vi "GM Count.vi"(0 "QUIT":refnum<vi>, 1 "Scan in Progress":refnum<vi>, 2 "GM1 Measure":refnum<vi>, 3 "Error":refnum<vi>, 4 "Measure GM2":refnum<vi>, 5 "VA Volts":refnum<vi>, 6 "VB Volts":refnum<vi>, 7 "Set Voltage A":refnum<vi>, 8 "GM1 Dwell":refnum<vi>, 9 "Set Voltage B":refnum<vi>, 10 "GM1 LLD":refnum<vi>, 12 "GM1 ULD":refnum<vi>, 14 "GM1 Counts":refnum<vi>, 16 "Emergency":refnum<vi>, 18 "GM2 Dwell":refnum<vi>, 20 "GM2 Counts":refnum<vi>) -> ()   [LabVIEW 2018]
uses:
  <vilib>/Utility/error.llb/DialogType.ctl
  <vilib>/Analysis/baseanly.llb/Mean (DBL).vi
  <vilib>/Analysis/NI_AALBase.lvlib
panel:
  out "Data":u32[](graph)
  out "GM2 Storage":dbl[](array[numeric])
  out "GM1 Storage":dbl[](array[numeric])
  in  "GM Count":T1(tab)
  out "Status B LED":bool
  out "Status A LED":bool
  in  "VB Local":dbl
  out "VB Feedback":dbl caption="(V)"
  out "VA Feedback":dbl caption="(V)"
  in  "VA Local":dbl caption="(V)"
  in  "GM2 Dwell Local":dbl=1.0 caption="Dwell" min=0.1
  in  "GM1 ULD":dbl caption="Upper Limit" max=12.0
  in  "GM1 Dwell Local":dbl=1.0 caption="Dwell" min=0.1
  in  "LLD Right":dbl caption="Lower Limit" max=12.0
  in  "GM2 Threshold":dbl caption="Threshold" min=0.0 max=10000.0 step=10.0
  in  "GM1 Threshold":dbl caption="Threshold" min=0.0 max=10000.0 step=10.0
  out "GM2 Counts Local":i32 caption="Total Counts"
  out "GM2 Rate":dbl caption="Count Rate"
  out "GM2 Average":dbl caption="Average Rate"
  out "Status A":string caption="Device Status Response"
  out "Status B":string caption="Device Status Response"
  out "GM1 Counts Local":i32 caption="Total Counts"
  out "GM1 Rate":dbl caption="Count Rate"
  out "GM1 Average":dbl caption="Average Rate"
  in  "Voltage Error Tolerance":dbl=2.0 caption="V"
  in  "Wait Time":dbl=10.0 caption="s"
  in  "VA Ramp":dbl=30.0 caption="A" min=2.0 step=1.0
  in  "Number of Rates\nto Average":u32=20 min=1 max=1024
  in  "GM1 Spectrum":i32=2 caption="Detector 1"
  in  "GM2 Spectrum":i32=3 caption="Detector 2"
  in  "NHQ 203M Voltage Supply":refnum<visa-resource-name>="COM8"
  out "VA Ramp Feedback":dbl=2.0 caption="V/s" format="%.2f"
  out "Voltage Change Response A":string caption="Voltage Change Response"
  out "Voltage Change Response B":string
  out "VB Ramp Feedback":dbl=2.0 caption="V/s" format="%.2f"
  in  "VB Ramp":sgl=30.0 caption="B" min=2 max=255 step=1
  in  "Feedback Delay":u32=50
  # "Note that the Average Rate is found by simply averaging the last 'n' acquired count rates.  Therefore,\nit may not be an accurate measure of the real count rate in Hz if Dwell has recently been changed."
  # "Detector 1"
  # "Detector 2"
  # "s"
  # "s"
  # "Hz"
  # "Hz"
  # "V"
  # "Hz"
  # "V"
  # "Hz"
  # "mV"
  # "mV"
  # "Voltage Supply B"
  # "Voltage Supply A"
  # "A"
  # "B"
  # "MCA 4 Spectrum #"
  # "NHQ 203 M Ramp Speed"
  # "Sometimes the power supply has trouble getting the actual voltage to the setpoint, especially for low voltages.  This can risk hanging up a scan, which waits for the voltage to reach the setpoint before allowing the next step to occur.  To avoid this problem, the VI will progress the scan if the difference between the actual voltage and the setpoint is less than <Voltage Error Tolerance> AND <Wait Time> has elapsed."
  # "The VI waits for <Feedback Delay> ms between submitting the change voltage command and then checking the state of the power supply."
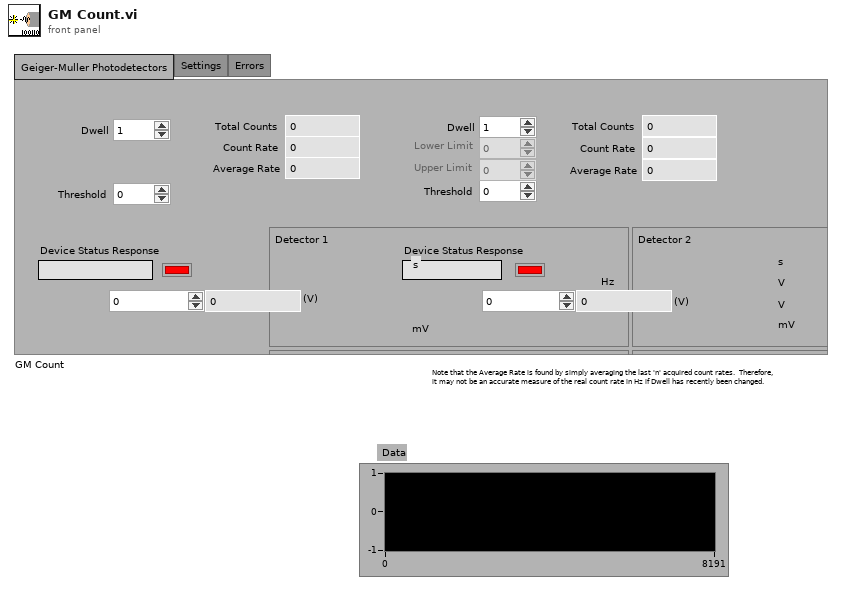
[diagram p1: front panel]
types:
  T1 = enum32{"Geiger-Muller Photodetectors", "Settings", "Errors"}
  T2 = typedef "DialogType.ctl" = u16
  T3 = typedef "iseg NHQ VISA Control.ctl" = cluster{"VISA Resource Name":refnum<visa-resource-name>, "FP Notation":bool, "Maximum Voltage":u32, "Maximum Current":u32}
  T4 = cluster{"Started":u32, "Maxval":u32, "Livetime":dbl, "Deadtime (%)":dbl, "Totalsum":dbl, "ROIsum":dbl, "ROIrate":dbl, "Realtime":dbl, "Netsum":dbl, "Counts":dbl}
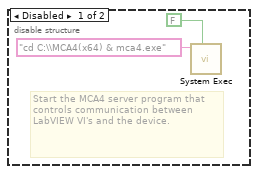
[diagram p2: hidden frame]
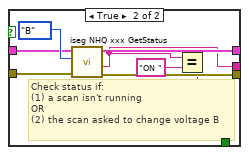
[diagram p5: hidden frame]
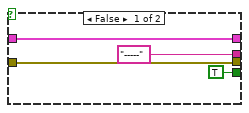
[diagram p6: hidden frame]
diagram:
  n1 = flat-sequence {
    frame #0 {
      w1 = FALSE ("Visible")
      # "GM1 = Right Detector\nGM2 = Left Detector"
      # "Initialize variables"
      n2 = disable-structure shown="Enabled" {
        frame Disabled {
          # "Start the MCA4 server program that controls communication between LabVIEW VI's and the device."
          n3 = call <vilib>:"System Exec.vi"("wait until completion? (T)"=FALSE, "command line"="cd C:\\MCA4(x64) & mca4.exe") -> ()  [unwired: 6 in, 4 out]
        }
        frame Enabled {
        }
      }
      n4 = Initialize Array(0.0 ("element"), 0 ("dimension size")) -> (→"GM1 Storage":dbl[])
      n5 = property on="GM1 Average" class="DigNum (strict)"("Value"=0.0 ("Average Right")) -> ()  [unwired: 2 in, 2 out]
      n6 = Initialize Array(0.0 ("element"), 0 ("dimension size")) -> (→"GM2 Storage":dbl[])
      n7 = property on="Set Voltage B" class="LVObjRef (strict)"("Visible"=w1) -> ()  [unwired: 2 in, 2 out]
      n8 = property on="QUIT" class="LVObjRef (strict)"("Visible"=w1) -> ()  [unwired: 2 in, 2 out]
      n9 = property on="GM1 Measure" class="LVObjRef (strict)"("Visible"=w1) -> ()  [unwired: 2 in, 2 out]
      n10 = property on="GM1 LLD" class="LVObjRef (strict)"("Visible"=w1) -> ()  [unwired: 2 in, 2 out]
      n11 = property on="Error" class="LVObjRef (strict)"("Visible"=w1) -> ()  [unwired: 2 in, 2 out]
      n12 = property on="GM1 ULD" class="LVObjRef (strict)"("Visible"=w1) -> ()  [unwired: 2 in, 2 out]
      n13 = property on="Scan in Progress" class="LVObjRef (strict)"("Visible"=w1) -> ()  [unwired: 2 in, 2 out]
      n14 = property on="GM1 Dwell" class="LVObjRef (strict)"("Visible"=w1) -> ()  [unwired: 2 in, 2 out]
      n15 = property on="GM1 Counts" class="LVObjRef (strict)"("Visible"=w1) -> ()  [unwired: 2 in, 2 out]
      n16 = property on="GM1 Storage" class="Arr (strict)"("Visible"=w1) -> ()  [unwired: 2 in, 2 out]
      n17 = property on="Measure GM2" class="LVObjRef (strict)"("Visible"=w1) -> ()  [unwired: 2 in, 2 out]
      n18 = property on="VB Volts" class="LVObjRef (strict)"("Visible"=w1) -> ()  [unwired: 2 in, 2 out]
      n19 = property on="VA Volts" class="LVObjRef (strict)"("Visible"=w1) -> ()  [unwired: 2 in, 2 out]
      n20 = property on="Set Voltage A" class="LVObjRef (strict)"("Visible"=w1) -> ()  [unwired: 2 in, 2 out]
    }
    frame #1 {
      n21 = while {
        stop <- w27 stop-if-true
        n22 = property on="Property Node" class="Bool (strict)"(reference="QUIT") -> ("Value"=w27:bool)  [unwired: 1 in, 2 out]
        n23 = property on="Property Node" class="Bool (strict)"(reference="Scan in Progress") -> ("Value"=w25:bool)  [unwired: 1 in, 2 out]
        n24 = property class="Bool (strict)"(reference="Set Voltage A") -> ("Value"=w15:bool)  [unwired: 1 in, 2 out]
        n25 = property class="Bool (strict)"(reference="Set Voltage B") -> ("Value"=w12:bool)  [unwired: 1 in, 2 out]
        n26 = property on="Property Node" class="Bool (strict)"(reference="GM1 Measure") -> ("Value"=w21:bool)  [unwired: 1 in, 2 out]
        n27 = property on="Property Node" class="Bool (strict)"(reference="Measure GM2") -> ("Value"=w18:bool)  [unwired: 1 in, 2 out]
        n28 = Not(x=w25) -> (.not. x?=w13:bool)
        n29 = Compound Arithmetic op=OR(w13, w15, w12) -> (w16:bool)
        n30 = Or(x=w13, y=w21) -> (x .or. y?=w20:bool)
        n31 = Or(x=w13, y=w15) -> (x .or. y?=w14:bool)
        n32 = Or(x=w13, y=w18) -> (x .or. y?=w19:bool)
        n33 = Or(x=w13, y=w12) -> (x .or. y?=w11:bool)
        n34 = case shown="True" w16 {
          tunnel: w14 -> [_ w30]
          tunnel: w11 -> [_ w29]
          frame False {
          }
          frame True {
            # "Talk to the voltage supply if:\n(1) there isn't a scan running\nOR\n(2) the scan has asked to set either voltage"
            n35 = flat-sequence {
              tunnel: "NHQ 203M Voltage Supply" -> [w42]
              tunnel: w30 -> [w41]
              tunnel: w29 -> [w40]
              frame #0 {
                # "Update global variables using\nlocal variables if a scan isn't\nrunning."
                n36 = property on="Scan in Progress" class="LVObjRef (strict)"() -> ("Value"=w33:refnum<vi>)  [unwired: 2 in, 2 out]
                n37 = property class="Bool (strict)"(reference=w33) -> ("Value"=w32:bool)  [unwired: 1 in, 2 out]
                n38 = case shown="False" w32 {
                  frame False {
                    n39 = property class="DigNum (strict)"(reference="VA Volts", "Value"="VA Local") -> ()  [unwired: 1 in, 2 out]
                    n40 = property class="DigNum (strict)"(reference="VB Volts", "Value"="VB Local") -> ()  [unwired: 1 in, 2 out]
                  }
                  frame True {
                  }
                }
              }
              frame #1 {
                n41 = Get Date/Time In Seconds() -> (seconds since 1Jan1904=w39:timestamp)
                n42 = To Double Precision Float(number=w39) -> (double precision float=w38:dbl)
                n43 = while {
                  tunnel: w42 -> [w117]
                  tunnel: w41 -> [w79]
                  tunnel: w40 -> [w78]
                  tunnel: w38 -> [w63]
                  stop <- w45 stop-if-true
                  w76 = T2 0 items=["no dialog", "OK message", "continue or stop message", "OK message + warnings", "continue/stop + warnings"] ("type of dialog (OK msg:1)")
                  # "Note the trailing space: \"ON \""
                  # "Repeat this procedure until:\n( (Nominal Voltage A = Voltage Feedback A)\nAND\n(Nominal Voltage B = Voltage Feeback B)\nAND\n( (Device Status A = \"ON \" )\nOR\n(Scan didn't ask to change Voltage A) )\nAND\n( (Device Status B = \"ON \" ) \nOR\n(Scan didn't ask to change Voltage B) ) )\nOR\n(A Scan is NOT Running)\nOR\n(Emergency Stop)"
                  # "-Initialize RS232 connection\n-Set nominal voltage A (V)\n-Set nominal voltage B (V)\n-Set voltage ramp speed A (V/s)\n-Set voltage ramp speed B (V/s)\n-Start voltage change A; get string feedback\n-Start voltage change B; get string feedback\n-Read voltage ramp speed A (V/s)\n-Read voltage ramp speed B (V/s)\n-Read device status A as a string\n-Read device status B as a string\n-Read voltage A (V)\n-Read voltage B (V)\n-Close connection"
                  n44 = property on="VA Volts" class="LVObjRef (strict)"() -> ("Value"=w81:refnum<vi>)  [unwired: 2 in, 2 out]
                  n45 = Add(x=w63, y="Wait Time") -> (x+y=w60:dbl)
                  n46 = property on="VB Volts" class="LVObjRef (strict)"() -> ("Value"=w80:refnum<vi>)  [unwired: 2 in, 2 out]
                  n47 = property class="DigNum (strict)"(reference=w81) -> ("Value"=w68:dbl)  [unwired: 1 in, 2 out]
                  n48 = property class="DigNum (strict)"(reference=w80) -> ("Value"=w55:dbl)  [unwired: 1 in, 2 out]
                  n49 = call "iseg NHQ xxx Initialize.vi"("VISA resource name"=w117) -> ("VISA Session Out"=w127:T3, "error out"=w108:errorcluster)  [unwired: 13 in]
                  n50 = call "iseg NHQ xxx SetNominalVoltage.vi"("error in (no error)"=w108, "Voltage (0 V)"=w68, "Channel (A)"=enum16{"A", "B"}."A", "VISA Session"=w127) -> ("error out"=w106:errorcluster, "VISA Session Out"=w107:T3)  [unwired: 6 in]
                  n51 = call "iseg NHQ xxx SetNominalVoltage.vi"("error in (no error)"=w106, "Voltage (0 V)"=w55, "Channel (A)"=enum16{"A", "B"}."B", "VISA Session"=w107) -> ("error out"=w104:errorcluster, "VISA Session Out"=w105:T3)  [unwired: 6 in]
                  n52 = call "iseg NHQ xxx SetVoltageRamp.vi"("error in (no error)"=w104, "Voltage Ramp (2 V/s)"="VA Ramp", "Channel (A)"=enum16{"A", "B"}."A", "VISA Session"=w105) -> ("error out"=w102:errorcluster, "VISA Session Out"=w103:T3)  [unwired: 6 in]
                  n53 = call "iseg NHQ xxx SetVoltageRamp.vi"("error in (no error)"=w102, "Voltage Ramp (2 V/s)"="VB Ramp", "Channel (A)"=enum16{"A", "B"}."B", "VISA Session"=w103) -> ("error out"=w98:errorcluster, "VISA Session Out"=w99:T3)  [unwired: 6 in]
                  n54 = call "iseg NHQ xxx StartVoltageChange.vi"("error in (no error)"=w98, "Channel (A)"=enum16{"A", "B"}."A", "VISA Session"=w99) -> ("error out"=w96:errorcluster, "Start Voltage Change Device Response"=→"Voltage Change Response A":string, "VISA Session Out"=w97:T3)  [unwired: 6 in]
                  n55 = call "iseg NHQ xxx StartVoltageChange.vi"("error in (no error)"=w96, "Channel (A)"=enum16{"A", "B"}."B", "VISA Session"=w97) -> ("error out"=w92:errorcluster, "Start Voltage Change Device Response"=→"Voltage Change Response B":string, "VISA Session Out"=w93:T3)  [unwired: 6 in]
                  n56 = call "iseg NHQ xxx GetVoltageRamp.vi"("error in (no error)"=w92, "Channel (A)"=enum16{"A", "B"}."A", "VISA session"=w93) -> ("error out"=w90:errorcluster, "Voltage Ramp (V/s)"=→"VA Ramp Feedback":dbl, "VISA Session Out"=w91:T3)  [unwired: 6 in]
                  n57 = call "iseg NHQ xxx GetVoltageRamp.vi"("error in (no error)"=w90, "Channel (A)"=enum16{"A", "B"}."B", "VISA session"=w91) -> ("error out"=w72:errorcluster, "Voltage Ramp (V/s)"=→"VB Ramp Feedback":dbl, "VISA Session Out"=w73:T3)  [unwired: 6 in]
                  n58 = flat-sequence {
                    tunnel: w73 -> [w133]
                    tunnel: w72 -> [w132]
                    tunnel: [w133] -> w71
                    tunnel: [w132] -> w70
                    frame #0 {
                      n59 = Wait (ms)(milliseconds to wait="Feedback Delay") -> ()  [unwired: 1 out]
                    }
                  }
                  n60 = case shown="True" w79 {
                    tunnel: ["-----" ("Device Status Response") w156] -> w123
                    tunnel: [w149 w155] -> w95
                    tunnel: [w148 w154] -> w94
                    tunnel: w71 -> [w149 w153]
                    tunnel: w70 -> [w148 w152]
                    tunnel: [TRUE w150] -> w75
                    frame False {
                    }
                    frame True {
                      # "Check status if:\n(1) a scan isn't running\nOR\n(2) the scan asked to change voltage A"
                      n61 = call "iseg NHQ xxx GetStatus.vi"("error in (no error)"=w152, "Channel (A)"=enum16{"A", "B"}."A", "VISA Session"=w153) -> ("error out"=w154:errorcluster, "Device Status Response"=w156:string, "VISA Session Out"=w155:T3)  [unwired: 6 in]
                      n62 = Equal?(x=w156, y="ON ") -> (x = y?=w150:bool)
                    }
                  }
                  "Status A" <- w123
                  n63 = case shown="False" w78 {
                    tunnel: w95 -> [w137 w144]
                    tunnel: w94 -> [w136 w143]
                    tunnel: [w137 w142] -> w87
                    tunnel: [w136 w141] -> w86
                    tunnel: ["-----" ("Device Status Response") w140] -> w83
                    tunnel: [TRUE w138] -> w74
                    frame False {
                    }
                    frame True {
                      # "Check status if:\n(1) a scan isn't running\nOR\n(2) the scan asked to change voltage B"
                      n64 = call "iseg NHQ xxx GetStatus.vi"("error in (no error)"=w143, "Channel (A)"=enum16{"A", "B"}."B", "VISA Session"=w144) -> ("error out"=w141:errorcluster, "Device Status Response"=w140:string, "VISA Session Out"=w142:T3)  [unwired: 6 in]
                      n65 = Equal?(x=w140, y="ON ") -> (x = y?=w138:bool)
                    }
                  }
                  "Status B" <- w83
                  n66 = Get Date/Time In Seconds() -> (seconds since 1Jan1904=w64:timestamp)
                  n67 = To Double Precision Float(number=w64) -> (double precision float=w61:dbl)
                  n68 = Greater?(x=w61, y=w60) -> (0:w49:bool)
                  n69 = call "iseg NHQ xxx GetActualVoltage.vi"("error in (no error)"=w86, "Channel (A)"=enum16{"A", "B"}."A", "VISA Session"=w87) -> ("error out"=w84:errorcluster, "Voltage"=w69:dbl, "VISA Session Out"=w85:T3)  [unwired: 5 in, 1 out]
                  "VA Feedback" <- w69
                  n70 = Equal?(x=w69, y=w68) -> (x = y?=w116:bool)
                  n71 = call "iseg NHQ xxx GetActualVoltage.vi"("error in (no error)"=w84, "Channel (A)"=enum16{"A", "B"}."B", "VISA Session"=w85) -> ("error out"=w114:errorcluster, "Voltage"=w54:dbl, "VISA Session Out"=w113:T3)  [unwired: 5 in, 1 out]
                  "VB Feedback" <- w54
                  n72 = Subtract(x=w55, y=w54) -> (x-y=w53:dbl)
                  n73 = Absolute Value(x=w53) -> (abs(x)=w52:dbl)
                  n74 = Less Or Equal?(x=w52, y="Voltage Error Tolerance") -> (x <= y?=w50:bool)
                  n75 = And(x=w50, y=w49) -> (x .and. y?=w48:bool)
                  n76 = Subtract(x=w69, y=w68) -> (x-y=w67:dbl)
                  n77 = And(x=w75, y=w116) -> (x .and. y?=w58:bool)
                  "Status A LED" <- w58
                  n78 = Absolute Value(x=w67) -> (abs(x)=w66:dbl)
                  n79 = call "iseg NHQ xxx Close.vi"("VISA session"=w113, "error in (no error)"=w114) -> ("error out"=w77:errorcluster)  [unwired: 13 in]
                  n80 = Equal?(x=w54, y=w55) -> (x = y?=w82:bool)
                  n81 = Less Or Equal?(x=w66, y="Voltage Error Tolerance") -> (x <= y?=w65:bool)
                  n82 = call <vilib>:"Simple Error Handler.vi"("type of dialog (OK msg:1)"=w76, "error in (no error)"=w77) -> ()  [unwired: 3 in, 5 out]
                  n83 = And(x=w74, y=w82) -> (x .and. y?=w56:bool)
                  "Status B LED" <- w56
                  n84 = And(x=w65, y=w49) -> (x .and. y?=w57:bool)
                  n85 = Or(x=w56, y=w48) -> (x .or. y?=w47:bool)
                  n86 = Or(x=w58, y=w57) -> (x .or. y?=w46:bool)
                  n87 = property on="Emergency" class="LVObjRef (strict)"() -> ("Value"=w115:refnum<vi>)  [unwired: 2 in, 2 out]
                  n88 = property on="Scan in Progress" class="LVObjRef (strict)"() -> ("Value"=w122:refnum<vi>)  [unwired: 2 in, 2 out]
                  n89 = property class="Bool (strict)"(reference=w115) -> ("Value"=w59:bool)  [unwired: 1 in, 2 out]
                  n90 = property class="Bool (strict)"(reference=w122) -> ("Value"=w121:bool)  [unwired: 1 in, 2 out]
                  n91 = And(x=w46, y=w47) -> (x .and. y?=w44:bool)
                  n92 = Not(x=w121) -> (.not. x?=w120:bool)
                  n93 = Or(x=w120, y=w59) -> (x .or. y?=w43:bool)
                  n94 = Or(x=w44, y=w43) -> (x .or. y?=w45:bool)
                }
              }
              frame #2 {
                w158 = FALSE ("Value")
                # "Tell the scan that voltages are done\nbeing set."
                n95 = property on="Set Voltage B" class="LVObjRef (strict)"() -> ("Value"=w159:refnum<vi>)  [unwired: 2 in, 2 out]
                n96 = property on="Set Voltage A" class="LVObjRef (strict)"() -> ("Value"=w160:refnum<vi>)  [unwired: 2 in, 2 out]
                n97 = property class="Bool (strict)"(reference=w160, "Value"=w158) -> ()  [unwired: 1 in, 2 out]
                n98 = property class="Bool (strict)"(reference=w159, "Value"=w158) -> ()  [unwired: 1 in, 2 out]
              }
            }
          }
        }
        n99 = case shown="True" w20 {
          frame False {
          }
          frame True {
            # "Take a measurement if\n(1) there isn't a scan running\nOR\n(2) there is a scan running and it has asked for a measurement"
            n100 = flat-sequence {
              tunnel: [w242] -> w225
              tunnel: w225 -> [w250]
              frame #0 {
                n101 = property on="Scan in Progress" class="LVObjRef (strict)"() -> ("Value"=w227:refnum<vi>)  [unwired: 2 in, 2 out]
                n102 = property on="Property Node" class="Bool (strict)"(reference=w227) -> ("Value"=w226:bool)  [unwired: 1 in, 2 out]
                n103 = case shown="False" w226 {
                  frame False {
                    # "Update some global variables if a scan isn't running"
                    n104 = property on="Property Node" class="DigNum (strict)"(reference="GM1 Dwell", "Value"="GM1 Dwell Local") -> ()  [unwired: 1 in, 2 out]
                  }
                  frame True {
                  }
                }
              }
              frame #1 {
                # "Set the minimum voltage that ADC1 will be sensitive to.  The MCA4 takes a 32 bit binary code.  The first 16 bits stay the same; the second indicate the voltage according to y=6*x+2852.\n(It may be more complicated than this.  See the manual for details.)"
                # "This sets the measurement dwell time, in seconds.\nUse \"rtpreset=\" for real time, or \"ltpreset=\"\nfor live time."
                # "This controls how the length of the\nmeasurement time is determined.\n1=real time\n2=live time (dead time corrected)\n4=event\n8=ROI\nSee manual for details"
                n105 = Multiply(x="GM1 Threshold", y=6.0) -> (x*y=w235:dbl)
                n106 = call "MC4Cmd.vi"("Command"="prena=1") -> ()  [unwired: 2 in, 1 out]
                n107 = Add(x=w235, y=2852.0) -> (x+y=w231:dbl)
                n108 = Add(x=186908672.0 ("y"), y=w231) -> (x+y=w233:dbl)
                n109 = Number To Decimal String(number=w233) -> (decimal integer string=w238:string)  [unwired: 1 in]
                n110 = property on="GM1 Spectrum" class="DigNum (strict)"() -> ("Value"=w241:i32)  [unwired: 2 in, 2 out]
                n111 = property on="GM1 Dwell" class="LVObjRef (strict)"() -> ("Value"=w245:refnum<vi>)  [unwired: 2 in, 2 out]
                n112 = Number To Decimal String(number=w241) -> (decimal integer string=w240:string)  [unwired: 1 in]
                n113 = property on="Property Node" class="DigNum (strict)"(reference=w245) -> ("Value"=w242:dbl)  [unwired: 1 in, 2 out]
                n114 = Concatenate Strings("thr", w240, "=" ("string"), w238) -> (w230:string)
                n115 = call "MC4Cmd.vi"("Command"=w230) -> ()  [unwired: 2 in, 1 out]
                n116 = Number To Decimal String(number=w242) -> (decimal integer string=w247:string)  [unwired: 1 in]
                n117 = Concatenate Strings("rtpreset=", w247) -> (w246:string)
                n118 = call "MC4Cmd.vi"("Command"=w246) -> ()  [unwired: 2 in, 1 out]
              }
              frame #2 {
                # "Take a measurement"
                n119 = call "MC4Cmd.vi"("Command"="start") -> ()  [unwired: 2 in, 1 out]
                n120 = Multiply(x=w250, y=900.0) -> (x*y=w251:dbl)
                n121 = Wait (ms)(milliseconds to wait=w251) -> ()  [unwired: 1 out]
              }
              frame #3 {
                # "Wait for the measurement to be done"
                n122 = while {
                  tunnel: ["GM1 Spectrum"] -> _
                  stop <- w259 stop-if-true
                  # "Get the current total count number"
                  # "Returns the status of the server as a digit.  Quit when it's idle."
                  n123 = call "MCA4MSts.vi"("Module #"=0) -> ("MStatus"=w265:cluster{"Running":u32, "Runtime":dbl})  [unwired: 1 in, 2 out]
                  n124 = call "MC4ADCSts.vi"("Spec #"="GM1 Spectrum") -> ("ADC Status"=w262:T4)  [unwired: 1 in, 1 out]
                  n125 = Unbundle(w265) -> ("Running"=w264:u32)  [unwired: 1 out]
                  n126 = Equal?(x=w264, y=u32 0) -> (x = y?=w258:bool)
                  n127 = Unbundle(w262) -> ("Realtime"=w254:dbl, "Counts"=w260:dbl)  [unwired: 8 out]
                  n128 = To Long Integer(number=w260) -> (32bit integer=→"GM1 Counts Local":i32)
                  n129 = Greater Than 0?(x=w254) -> (x > 0?=w255:bool)
                  n130 = property on="Property Node" class="Bool (strict)"(reference="Emergency") -> ("Value"=w256:bool)  [unwired: 1 in, 2 out]
                  n131 = case shown="True" w255 {
                    tunnel: w254 -> [_ w268]
                    tunnel: w260 -> [_ w267]
                    frame False {
                    }
                    frame True {
                      n132 = Divide(x=w267, y=w268) -> (x/y=→"GM1 Rate":dbl)
                    }
                  }
                  n133 = Or(x=w256, y=w258) -> (x .or. y?=w259:bool)
                }
              }
              frame #4 {
                # "Let the scan know that the measurement finished, if necessary"
                # "Do a final update of the results."
                n134 = property on="GM1 Spectrum" class="DigNum (strict)"() -> ("Value"=w272:i32)  [unwired: 2 in, 2 out]
                n135 = flat-sequence {
                  tunnel: [w283] -> w275
                  tunnel: w273 -> [w280]
                  tunnel: w275 -> [w287]
                  frame #0 {
                    # "Keep a record of recent count rates\nto average."
                    n136 = property on="GM1 Dwell" class="LVObjRef (strict)"() -> ("Value"=w279:refnum<vi>)  [unwired: 2 in, 2 out]
                    n137 = property on="GM1 Storage" class="Arr (strict)"() -> ("Value"=w284:dbl[])  [unwired: 2 in, 2 out]
                    n138 = property class="DigNum (strict)"(reference=w279) -> ("Value"=w278:dbl)  [unwired: 1 in, 2 out]
                    n139 = Divide(x=w280, y=w278) -> (x/y=w281:dbl)
                    n140 = Insert Into Array(array=w284, index=0, new element=w281) -> (w283:dbl[])
                    n141 = property on="GM1 Storage" class="Arr (strict)"("Value"=w283) -> ()  [unwired: 2 in, 2 out]
                  }
                  frame #1 {
                    # "If the storage array is longer than the number of\nrates to average, then remove old entries."
                    n142 = Array Size(array=w287) -> (size(s)=w286:i32)
                    n143 = Greater?(x=w286, y="Number of Rates\nto Average") -> (0:w288:bool)
                    n144 = case shown="True" w288 {
                      tunnel: w287 -> [_ w294]
                      tunnel: "Number of Rates\nto Average" -> [_ w292]
                      tunnel: w286 -> [_ w291]
                      tunnel: "Number of Rates\nto Average" -> [_ w290]
                      frame False {
                      }
                      frame True {
                        n145 = Subtract(x=w291, y=w290) -> (x-y=w289:u32)
                        n146 = Delete From Array(array=w294, length=w289, index=w292) -> (array with subset deleted=w293:dbl[])  [unwired: 1 out]
                        n147 = property on="GM1 Storage" class="Arr (strict)"("Value"=w293) -> ()  [unwired: 2 in, 2 out]
                      }
                    }
                  }
                  frame #2 {
                    # "Calculate the average."
                    n148 = property on="GM1 Storage" class="Arr (strict)"() -> ("Value"=w296:dbl[])  [unwired: 2 in, 2 out]
                    n149 = call-poly <vilib>:"Mean.vi"("X"=w296) -> ("mean"=→"GM1 Average":dbl)  [unwired: 1 out]
                  }
                }
                n150 = call "MC4ADCSts.vi"("Spec #"=w272) -> ("ADC Status"=w277:T4)  [unwired: 1 in, 1 out]
                n151 = Unbundle(w277) -> ("Counts"=w276:dbl)  [unwired: 9 out]
                n152 = To Long Integer(number=w276) -> (32bit integer=w273:i32)
                n153 = property on="GM1 Counts Local" class="DigNum (strict)"("Value"=w273) -> ()  [unwired: 2 in, 2 out]
                n154 = property class="DigNum (strict)"(reference="GM1 Counts", "Value"=w273) -> ()  [unwired: 1 in, 2 out]
                n155 = property on="GM1 Measure" class="LVObjRef (strict)"() -> ("Value"=w271:refnum<vi>)  [unwired: 2 in, 2 out]
                n156 = property class="Bool (strict)"(reference=w271, "Value"=FALSE) -> ()  [unwired: 1 in, 2 out]
              }
            }
          }
        }
        n157 = case shown="True" w19 {
          frame False {
          }
          frame True {
            n158 = flat-sequence {
              tunnel: [w170] -> w161
              tunnel: w161 -> [w180]
              frame #0 {
                n159 = property on="Scan in Progress" class="LVObjRef (strict)"() -> ("Value"=w163:refnum<vi>)  [unwired: 2 in, 2 out]
                n160 = property class="Bool (strict)"(reference=w163) -> ("Value"=w162:bool)  [unwired: 1 in, 2 out]
                n161 = case shown="False" w162 {
                  frame False {
                    n162 = property class="DigNum (strict)"(reference="GM2 Dwell", "Value"="GM2 Dwell Local") -> ()  [unwired: 1 in, 2 out]
                  }
                  frame True {
                  }
                }
              }
              frame #1 {
                (unwired) 6.0 ("y")
                (unwired) 186908672.0 ("y")
                (unwired) 2852.0 ("y")
                n163 = call "MC4Cmd.vi"("Command"="prena=1") -> ()  [unwired: 2 in, 1 out]
                n164 = property on="GM2 Spectrum" class="DigNum (strict)"() -> ("Value"=w169:i32)  [unwired: 2 in, 2 out]
                n165 = Number To Hexadecimal String(2:"GM2 Threshold") -> (0:w167:string)  [unwired: 1 in]
                n166 = Number To Decimal String(number=w169) -> (decimal integer string=w176:string)  [unwired: 1 in]
                n167 = property on="GM2 Dwell" class="LVObjRef (strict)"() -> ("Value"=w174:refnum<vi>)  [unwired: 2 in, 2 out]
                n168 = Concatenate Strings("thr", w176, "=" ("string"), w167) -> ()  [unwired: 1 out]
                n169 = property class="DigNum (strict)"(reference=w174) -> ("Value"=w170:dbl)  [unwired: 1 in, 2 out]
                n170 = Number To Decimal String(number=w170) -> (decimal integer string=w173:string)  [unwired: 1 in]
                n171 = Concatenate Strings("rtpreset=", w173) -> (w172:string)
                n172 = call "MC4Cmd.vi"("Command"=w172) -> ()  [unwired: 2 in, 1 out]
              }
              frame #2 {
                n173 = Multiply(x=w180, y=900.0) -> (x*y=w179:dbl)
                n174 = Wait (ms)(milliseconds to wait=w179) -> ()  [unwired: 1 out]
                n175 = call "MC4Cmd.vi"("Command"="start") -> ()  [unwired: 2 in, 1 out]
              }
              frame #3 {
                n176 = while {
                  stop <- w193 stop-if-true
                  n177 = call "MC4ADCSts.vi"("Spec #"="GM2 Spectrum") -> ("ADC Status"=w187:T4)  [unwired: 1 in, 1 out]
                  n178 = call "MCA4MSts.vi"("Module #"=0) -> ("MStatus"=w190:cluster{"Running":u32, "Runtime":dbl})  [unwired: 1 in, 2 out]
                  n179 = Unbundle(w187) -> ("Realtime"=w183:dbl, "Counts"=w184:dbl)  [unwired: 8 out]
                  n180 = Unbundle(w190) -> ("Running"=w189:u32)  [unwired: 1 out]
                  n181 = To Long Integer(number=w184) -> (32bit integer=→"GM2 Counts Local":i32)
                  n182 = Equal To 0?(x=w189) -> (x = 0?=w188:bool)
                  n183 = property on="Emergency" class="LVObjRef (strict)"() -> ("Value"=w194:refnum<vi>)  [unwired: 2 in, 2 out]
                  n184 = Greater Than 0?(x=w183) -> (x > 0?=w185:bool)
                  n185 = property class="Bool (strict)"(reference=w194) -> ("Value"=w192:bool)  [unwired: 1 in, 2 out]
                  n186 = case shown="True" w185 {
                    tunnel: w184 -> [_ w197]
                    tunnel: w183 -> [_ w196]
                    frame False {
                    }
                    frame True {
                      n187 = Divide(x=w197, y=w196) -> (x/y=→"GM2 Rate":dbl)
                    }
                  }
                  n188 = Or(x=w192, y=w188) -> (x .or. y?=w193:bool)
                }
              }
              frame #4 {
                n189 = property on="GM2 Spectrum" class="DigNum (strict)"() -> ("Value"=w199:i32)  [unwired: 2 in, 2 out]
                n190 = call "MC4Dat.vi"("Spectrum #"=w199) -> ("Data"=→"Data":u32[])  [unwired: 2 in, 2 out]
                n191 = call "MC4ADCSts.vi"("Spec #"=w199) -> ("ADC Status"=w206:T4)  [unwired: 1 in, 1 out]
                n192 = property on="Measure GM2" class="LVObjRef (strict)"() -> ("Value"=w200:refnum<vi>)  [unwired: 2 in, 2 out]
                n193 = Unbundle(w206) -> ("Counts"=w203:dbl)  [unwired: 9 out]
                n194 = To Long Integer(number=w203) -> (32bit integer=w204:i32)
                n195 = property class="Bool (strict)"(reference=w200, "Value"=FALSE) -> ()  [unwired: 1 in, 2 out]
                n196 = property on="GM2 Counts Local" class="DigNum (strict)"("Value"=w204) -> ()  [unwired: 2 in, 2 out]
                n197 = property class="DigNum (strict)"(reference="GM2 Counts", "Value"=w204) -> ()  [unwired: 1 in, 2 out]
                n198 = flat-sequence {
                  tunnel: w203 -> [w211]
                  tunnel: [w207] -> w202
                  tunnel: w202 -> [w216]
                  frame #0 {
                    n199 = property on="GM2 Dwell" class="LVObjRef (strict)"() -> ("Value"=w213:refnum<vi>)  [unwired: 2 in, 2 out]
                    n200 = property class="DigNum (strict)"(reference=w213) -> ("Value"=w212:dbl)  [unwired: 1 in, 2 out]
                    n201 = Divide(x=w211, y=w212) -> (x/y=w209:dbl)
                    n202 = property on="GM2 Storage" class="Arr (strict)"() -> ("Value"=w210:dbl[])  [unwired: 2 in, 2 out]
                    n203 = Insert Into Array(array=w210, index=0, new element=w209) -> (w207:dbl[])
                    n204 = property on="GM2 Storage" class="Arr (strict)"("Value"=w207) -> ()  [unwired: 2 in, 2 out]
                  }
                  frame #1 {
                    n205 = property on="Number of Rates\nto Average" class="DigNum (strict)"() -> ("Value"=w215:u32)  [unwired: 2 in, 2 out]
                    n206 = Array Size(array=w216) -> (size(s)=w214:i32)
                    n207 = Greater?(x=w214, y=w215) -> (0:w217:bool)
                    n208 = case shown="True" w217 {
                      tunnel: w216 -> [_ w222]
                      tunnel: w215 -> [_ w219]
                      tunnel: w214 -> [_ w220]
                      frame False {
                      }
                      frame True {
                        n209 = Subtract(x=w220, y=w219) -> (x-y=w221:u32)
                        n210 = Delete From Array(array=w222, length=w221, index=w219) -> (array with subset deleted=w218:dbl[])  [unwired: 1 out]
                        n211 = property on="GM2 Storage" class="Arr (strict)"("Value"=w218) -> ()  [unwired: 2 in, 2 out]
                      }
                    }
                  }
                  frame #2 {
                    n212 = property on="GM2 Storage" class="Arr (strict)"() -> ("Value"=w224:dbl[])  [unwired: 2 in, 2 out]
                    n213 = call-poly <vilib>:"Mean.vi"("X"=w224) -> ("mean"=→"GM2 Average":dbl)  [unwired: 1 out]
                  }
                }
              }
            }
          }
        }
      }
    }
  }
